vi "R4DataCollection.vi"(8 "error constant":errorcluster, 10 "Write Once":bool, 11 "LabVIEW Web Service":refnum<class "Web Service.lvclass">) -> (0 "error out":errorcluster={"status"=FALSE, "code"=0, "source"="0"})   [LabVIEW 2016]
uses:
  <vilib>/wsapi/Web Service.lvclass
  <vilib>/Platform/TimedLoop/XDataNode/timing_clust.ctl
  <vilib>/Platform/TimedLoop/XDataNode/nitl_modes.ctl
  <vilib>/Platform/TimedLoop/XDataNode/wakeup.ctl
  <vilib>/Platform/TimedLoop/XDataNode/XDataNode.xnode
  <vilib>/Platform/TimedLoop/XDataNode/XDNodeRunTimeDep.lvlib
  <vilib>/ptbypt/NI_PtbyPt.lvlib
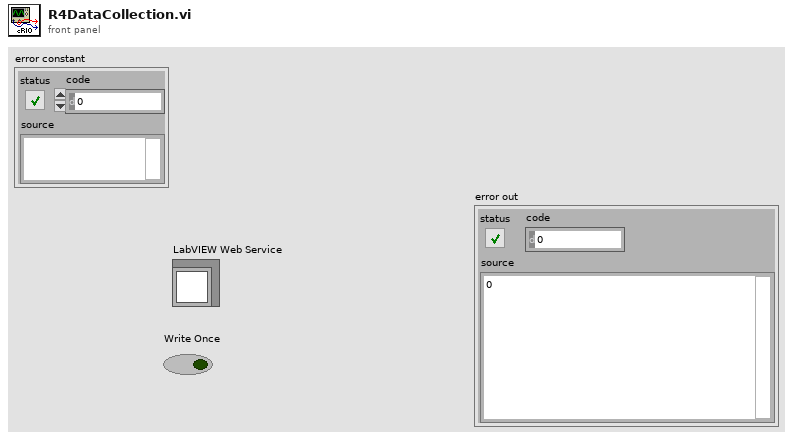
[diagram p1: front panel]
types:
  T1 = typedef "XDNodeRunTimeDep.lvlib/timing_clust.ctl" = cluster{"Expected End [f-1]":u64, "Actual End [f-1]":u64, "Finished Late? [f-1]":bool, "Expected End [i-1]":u64, "Actual End [i-1]":u64, "Finished Late? [i-1]":bool, "Expected Start [i]":u64, "Actual Start [i]":u64, "Expected Start [f]":u64, "Actual Start [f]":u64, "Source Name":string, "Structure Name":string, "Period":i64, "Deadline":i64, "Offset":i64, "Start":i64, "Priority":i32, "Timeout":i32, "Mode":T2, "Wakeup Reason":T3, "Error":errorcluster, "Source Type":string, "Secondary Source Type":string, "Global End Time":u64, "Global Start Time":u64, "Frame Duration":u64, "Iteration Duration":u64, "Assigned CPU":i32, "I/O Scan Engine Mode":u32}
  T2 = typedef "XDNodeRunTimeDep.lvlib/nitl_modes.ctl" = enum32{"No Change", "Process missed periods, maintain original phase", "Discard missed periods, maintain original phase", "Process missed periods, ignore original phase", "Discard missed periods, ignore original phase"}
  T3 = typedef "XDNodeRunTimeDep.lvlib/wakeup.ctl" = enum32{"Normal", "Aborted", "Asynchronous wakeup", "Timing source error", "Timed loop error", "Timeout"}
  T4 = cluster{"Media Pump":bool, "Water Pump":bool, "Gas Pump":bool, "Effluent Pump":bool, "Release Pump":bool}
  T5 = cluster{"Array of Double[0]":dbl, "Array of Double[1]":dbl, "Array of Double[2]":dbl, "Array of Double[3]":dbl, "Array of Double[4]":dbl, "Array of Double[5]":dbl, "Array of Double[6]":dbl, "Array of Double[7]":dbl, "Array of Double[8]":dbl}
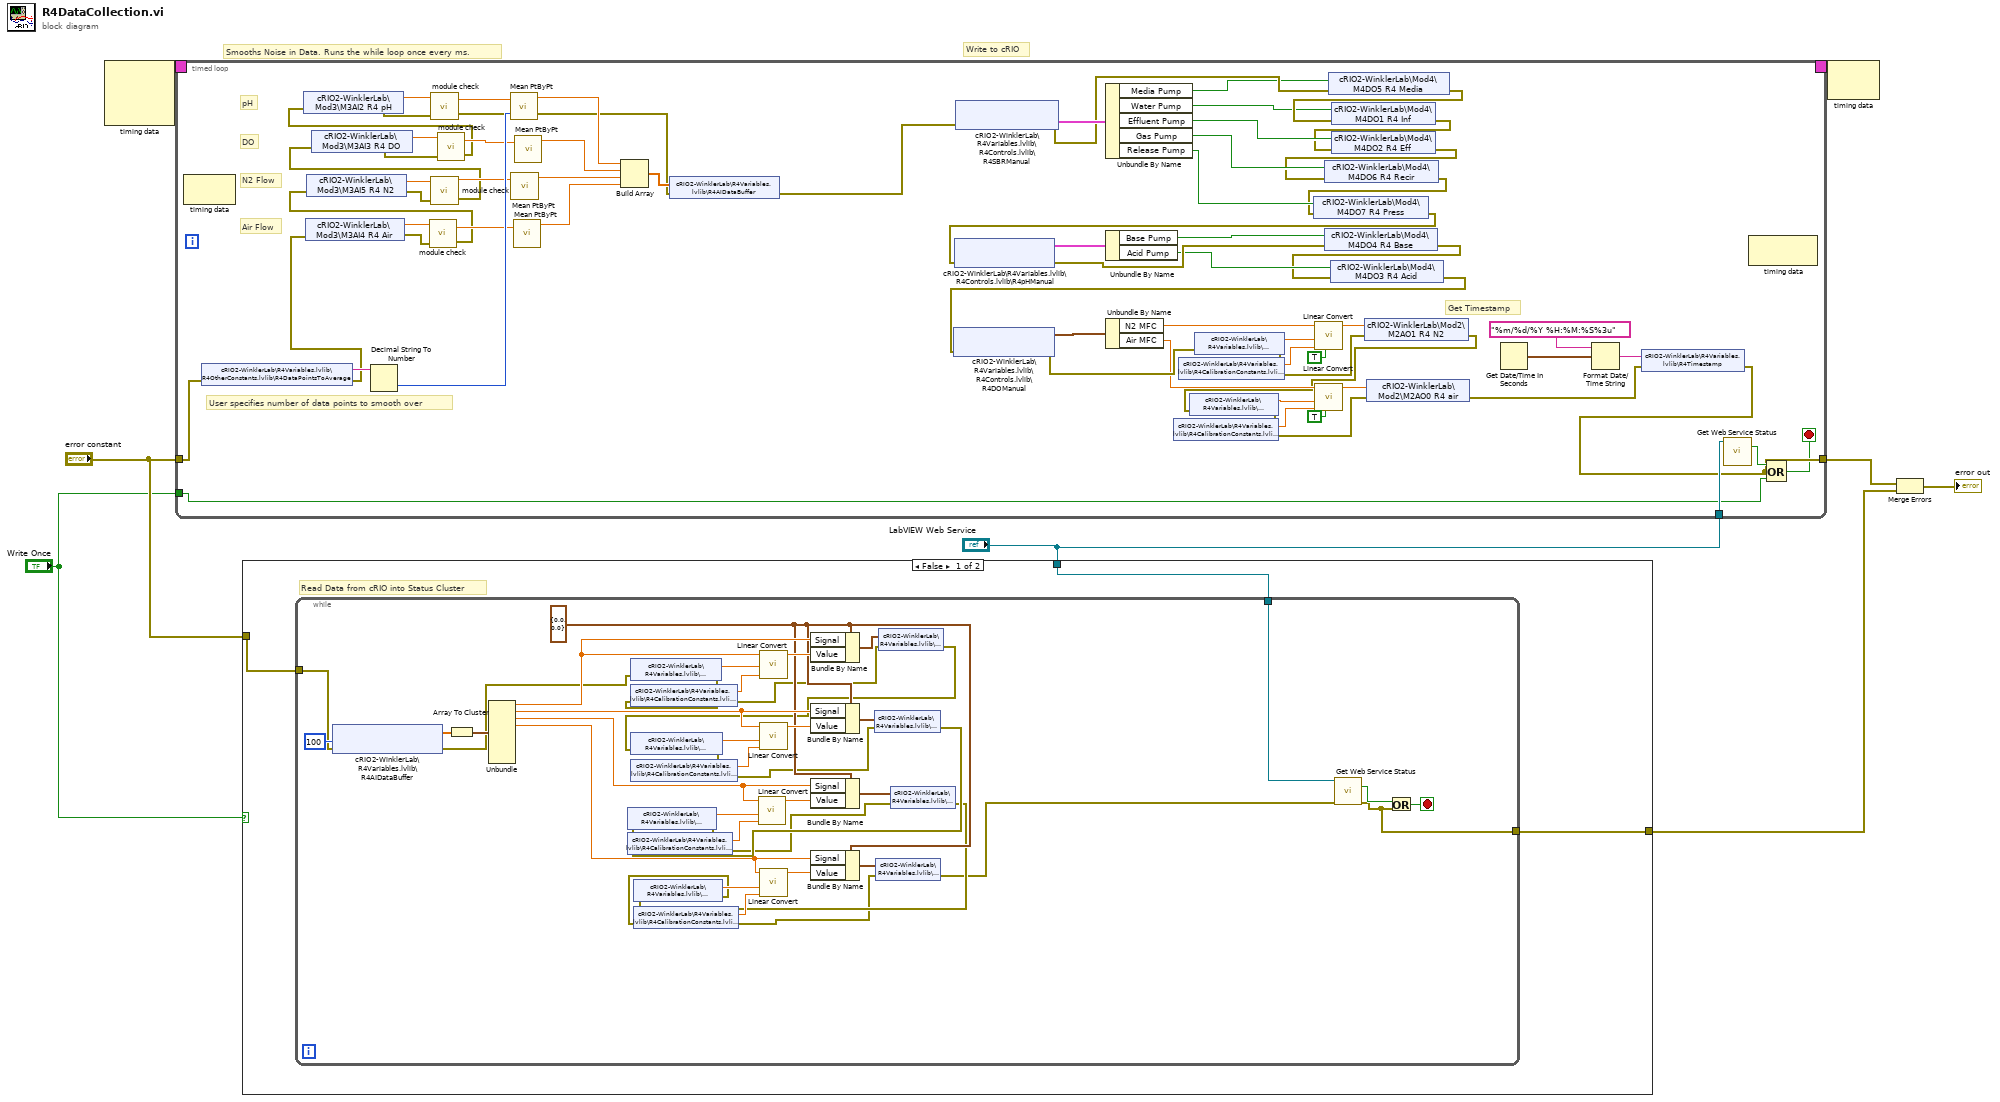
[diagram p0: block diagram]
diagram:
  # "Write to cRIO"
  # "Smooths Noise in Data. Runs the while loop once every ms."
  n1 = node-c288() -> (w8:T1)  [unwired: 3 in]
  n2 = timed-loop {
    timing: w8 -> [_]
    timing-out: [_] -> w7
    tunnel: "error constant" -> [w71]
    tunnel: "LabVIEW Web Service" -> [w67]
    tunnel: "Write Once" -> [w65]
    tunnel: [w64] -> w3
    stop <- w63 stop-if-true
    # "Get Timestamp"
    # "User specifies number of data points to smooth over"
    # "Air Flow"
    # "N2 Flow"
    # "DO"
    # "pH"
    n3 = node-c288() -> ()  [unwired: 1 in, 1 out]
    n4 = shared-variable "cRIO2-WinklerLab\\R4Variables.lvlib\\R4OtherConstants.lvlib\\R4DataPointsToAverage"(error in=w71) -> (w74:string, error out=w47:errorcluster)
    n5 = shared-variable "cRIO2-WinklerLab\\Mod3\\M3AI4 R4 Air"(error in=w47) -> (w13:dbl, error out=w12:errorcluster)
    n6 = Decimal String To Number(string=w74) -> (number=w62:i32)  [unwired: 2 in, 1 out]
    n7 = call "module check.vi"("error in"=w12, "Value"=w13) -> ("error constant"=w14:errorcluster, "Value out"=w15:dbl)  [unwired: 1 in]
    n8 = shared-variable "cRIO2-WinklerLab\\Mod3\\M3AI5 R4 N2"(error in=w14) -> (w17:dbl, error out=w16:errorcluster)
    n9 = call "module check.vi"("error in"=w16, "Value"=w17) -> ("error constant"=w18:errorcluster, "Value out"=w19:dbl)  [unwired: 1 in]
    n10 = shared-variable "cRIO2-WinklerLab\\Mod3\\M3AI3 R4 DO"(error in=w18) -> (w21:dbl, error out=w20:errorcluster)
    n11 = call "module check.vi"("error in"=w20, "Value"=w21) -> ("error constant"=w22:errorcluster, "Value out"=w23:dbl)  [unwired: 1 in]
    n12 = shared-variable "cRIO2-WinklerLab\\Mod3\\M3AI2 R4 pH"(error in=w22) -> (w26:dbl, error out=w24:errorcluster)
    n13 = call "module check.vi"("error in"=w24, "Value"=w26) -> ("error constant"=w25:errorcluster, "Value out"=w27:dbl)  [unwired: 1 in]
    n14 = call <vilib>:"Mean PtByPt.vi"("x"=w27, "sample length"=w62) -> ("mean"=w61:dbl)  [unwired: 2 in, 1 out]
    n15 = call <vilib>:"Mean PtByPt.vi"("x"=w19) -> ("mean"=w59:dbl)  [unwired: 3 in, 1 out]
    n16 = call <vilib>:"Mean PtByPt.vi"("x"=w15) -> ("mean"=w60:dbl)  [unwired: 3 in, 1 out]
    n17 = call <vilib>:"Mean PtByPt.vi"("x"=w23) -> ("mean"=w58:dbl)  [unwired: 3 in, 1 out]
    n18 = Build Array(w61, w58, w59, w60) -> (w78:dbl[])
    n19 = shared-variable "cRIO2-WinklerLab\\R4Variables.lvlib\\R4AIDataBuffer"(w78, error in=w25) -> (error out=w70:errorcluster)
    n20 = shared-variable "cRIO2-WinklerLab\\R4Variables.lvlib\\R4Controls.lvlib\\R4SBRManual"(error in=w70) -> (w73:T4, error out=w46:errorcluster)  [unwired: 1 in, 1 out]
    n21 = Unbundle By Name(w73) -> ("Media Pump"=w45:bool, "Water Pump"=w43:bool, "Effluent Pump"=w42:bool, "Gas Pump"=w40:bool, "Release Pump"=w11:bool)
    n22 = shared-variable "cRIO2-WinklerLab\\Mod4\\M4DO5 R4 Media"(w45, error in=w46) -> (error out=w44:errorcluster)
    n23 = shared-variable "cRIO2-WinklerLab\\Mod4\\M4DO1 R4 Inf"(w43, error in=w44) -> (error out=w41:errorcluster)
    n24 = shared-variable "cRIO2-WinklerLab\\Mod4\\M4DO2 R4 Eff"(w42, error in=w41) -> (error out=w39:errorcluster)
    n25 = shared-variable "cRIO2-WinklerLab\\Mod4\\M4DO6 R4 Recir"(w40, error in=w39) -> (error out=w10:errorcluster)
    n26 = shared-variable "cRIO2-WinklerLab\\Mod4\\M4DO7 R4 Press"(w11, error in=w10) -> (error out=w9:errorcluster)
    n27 = shared-variable "cRIO2-WinklerLab\\R4Variables.lvlib\\R4Controls.lvlib\\R4pHManual"(error in=w9) -> (w72:cluster{"Acid Pump":bool, "Base Pump":bool}, error out=w37:errorcluster)  [unwired: 1 in, 1 out]
    n28 = Unbundle By Name(w72) -> ("Base Pump"=w38:bool, "Acid Pump"=w36:bool)
    n29 = shared-variable "cRIO2-WinklerLab\\Mod4\\M4DO4 R4 Base"(w38, error in=w37) -> (error out=w35:errorcluster)
    n30 = shared-variable "cRIO2-WinklerLab\\Mod4\\M4DO3 R4 Acid"(w36, error in=w35) -> (error out=w34:errorcluster)
    n31 = shared-variable "cRIO2-WinklerLab\\R4Variables.lvlib\\R4Controls.lvlib\\R4DOManual"(error in=w34) -> (w69:cluster{"Air MFC":dbl, "N2 MFC":dbl}, error out=w68:errorcluster)  [unwired: 1 in, 1 out]
    n32 = Unbundle By Name(w69) -> ("N2 MFC"=w57:dbl, "Air MFC"=w56:dbl)
    n33 = shared-variable "cRIO2-WinklerLab\\R4Variables.lvlib\\R4CalibrationConstants.lvlib\\R4N2Slope"(error in=w68) -> (w51:dbl, error out=w49:errorcluster)
    n34 = shared-variable "cRIO2-WinklerLab\\R4Variables.lvlib\\R4CalibrationConstants.lvlib\\R4N2Intercept"(error in=w49) -> (w50:dbl, error out=w30:errorcluster)
    n35 = call "Linear Convert.vi"("Inverse?"=TRUE, "Intercept"=w50, "Slope"=w51, "Signal"=w57) -> ("Result"=w29:dbl)  [unwired: 7 in]
    n36 = shared-variable "cRIO2-WinklerLab\\Mod2\\M2AO1 R4 N2"(w29, error in=w30) -> (error out=w28:errorcluster)
    n37 = shared-variable "cRIO2-WinklerLab\\R4Variables.lvlib\\R4CalibrationConstants.lvlib\\R4AirSlope"(error in=w28) -> (w53:dbl, error out=w48:errorcluster)
    n38 = shared-variable "cRIO2-WinklerLab\\R4Variables.lvlib\\R4CalibrationConstants.lvlib\\R4AirIntercept"(error in=w48) -> (w52:dbl, error out=w32:errorcluster)
    n39 = call "Linear Convert.vi"("Inverse?"=TRUE, "Intercept"=w52, "Slope"=w53, "Signal"=w56) -> ("Result"=w31:dbl)  [unwired: 7 in]
    n40 = shared-variable "cRIO2-WinklerLab\\Mod2\\M2AO0 R4 air"(w31, error in=w32) -> (error out=w33:errorcluster)
    n41 = Get Date/Time In Seconds() -> (seconds since 1Jan1904=w76:timestamp)
    n42 = Format Date/Time String(time format string (%c)="%m/%d/%Y %H:%M:%S%3u", seconds (now)=w76) -> (date/time string=w75:string)  [unwired: 1 in]
    n43 = shared-variable "cRIO2-WinklerLab\\R4Variables.lvlib\\R4Timestamp"(w75, error in=w33) -> (error out=w64:errorcluster)
    n44 = call <vilib>:"Get Web Service Status.vi"("LabVIEW Web Service"=w67) -> ("service stopping?"=w66:bool)  [unwired: 12 in, 2 out]
    n45 = node-c288() -> ()  [unwired: 1 in, 1 out]
    n46 = Compound Arithmetic op=OR(w66, w64, w65) -> (w63:bool)
  }
  n47 = case shown="False" "Write Once" {
    tunnel: "error constant" -> [w83 w126]
    tunnel: "LabVIEW Web Service" -> [w82 _]
    tunnel: [w81 w126] -> w2
    frame False {
      # "Read Data from cRIO into Status Cluster"
      n48 = while {
        tunnel: w83 -> [w90]
        tunnel: [w89] -> w81
        tunnel: w82 -> [w88]
        stop <- w116 stop-if-true
        w107 = cluster{"Signal":dbl, "Value":dbl} {"Signal"=0.0, "Value"=0.0} ("Analog Input")
        n49 = shared-variable "cRIO2-WinklerLab\\R4Variables.lvlib\\R4AIDataBuffer"(error in=w90, u32 100 ("milliseconds to wait")) -> (w123:dbl[], error out=w100:errorcluster)  [unwired: 1 out]
        n50 = Array To Cluster(array=w123) -> (cluster=w125:T5)
        n51 = Unbundle(w125) -> ("Array of Double[0]"=w121:dbl, "Array of Double[1]"=w120:dbl, "Array of Double[2]"=w109:dbl, "Array of Double[3]"=w108:dbl)  [unwired: 5 out]
        n52 = shared-variable "cRIO2-WinklerLab\\R4Variables.lvlib\\R4CalibrationConstants.lvlib\\R4pHSlope"(error in=w100) -> (w114:dbl, error out=w99:errorcluster)
        n53 = shared-variable "cRIO2-WinklerLab\\R4Variables.lvlib\\R4CalibrationConstants.lvlib\\R4pHIntercept"(error in=w99) -> (w115:dbl, error out=w85:errorcluster)
        n54 = call "Linear Convert.vi"("Intercept"=w115, "Slope"=w114, "Signal"=w121) -> ("Result"=w122:dbl)  [unwired: 8 in]
        n55 = Bundle By Name(cluster=w107, "Signal"=w121, "Value"=w122) -> (w86:cluster{"Signal":dbl, "Value":dbl})
        n56 = shared-variable "cRIO2-WinklerLab\\R4Variables.lvlib\\R4Signals.lvlib\\R4pH"(w86, error in=w85) -> (error out=w87:errorcluster)
        n57 = shared-variable "cRIO2-WinklerLab\\R4Variables.lvlib\\R4CalibrationConstants.lvlib\\R4DOSlope"(error in=w87) -> (w113:dbl, error out=w98:errorcluster)
        n58 = shared-variable "cRIO2-WinklerLab\\R4Variables.lvlib\\R4CalibrationConstants.lvlib\\R4DOIntercept"(error in=w98) -> (w112:dbl, error out=w97:errorcluster)
        n59 = call "Linear Convert.vi"("Intercept"=w112, "Slope"=w113, "Signal"=w120) -> ("Result"=w118:dbl)  [unwired: 8 in]
        n60 = Bundle By Name(cluster=w107, "Signal"=w120, "Value"=w118) -> (w119:cluster{"Signal":dbl, "Value":dbl})
        n61 = shared-variable "cRIO2-WinklerLab\\R4Variables.lvlib\\R4Signals.lvlib\\R4DO"(w119, error in=w97) -> (error out=w96:errorcluster)
        n62 = shared-variable "cRIO2-WinklerLab\\R4Variables.lvlib\\R4CalibrationConstants.lvlib\\R4N2Slope"(error in=w96) -> (w104:dbl, error out=w95:errorcluster)
        n63 = shared-variable "cRIO2-WinklerLab\\R4Variables.lvlib\\R4CalibrationConstants.lvlib\\R4N2Intercept"(error in=w95) -> (w103:dbl, error out=w94:errorcluster)
        n64 = call "Linear Convert.vi"("Intercept"=w103, "Slope"=w104, "Signal"=w109) -> ("Result"=w110:dbl)  [unwired: 8 in]
        n65 = Bundle By Name(cluster=w107, "Signal"=w109, "Value"=w110) -> (w101:cluster{"Signal":dbl, "Value":dbl})
        n66 = shared-variable "cRIO2-WinklerLab\\R4Variables.lvlib\\R4Signals.lvlib\\R4N2"(w101, error in=w94) -> (error out=w93:errorcluster)
        n67 = shared-variable "cRIO2-WinklerLab\\R4Variables.lvlib\\R4CalibrationConstants.lvlib\\R4AirSlope"(error in=w93) -> (w106:dbl, error out=w92:errorcluster)
        n68 = shared-variable "cRIO2-WinklerLab\\R4Variables.lvlib\\R4CalibrationConstants.lvlib\\R4AirIntercept"(error in=w92) -> (w105:dbl, error out=w91:errorcluster)
        n69 = call "Linear Convert.vi"("Intercept"=w105, "Slope"=w106, "Signal"=w108) -> ("Result"=w111:dbl)  [unwired: 8 in]
        n70 = Bundle By Name(cluster=w107, "Signal"=w108, "Value"=w111) -> (w102:cluster{"Signal":dbl, "Value":dbl})
        n71 = shared-variable "cRIO2-WinklerLab\\R4Variables.lvlib\\R4Signals.lvlib\\R4Air"(w102, error in=w91) -> (error out=w84:errorcluster)
        n72 = call <vilib>:"Get Web Service Status.vi"("LabVIEW Web Service"=w88, "error in (no error)"=w84) -> ("service stopping?"=w117:bool, "error out"=w89:errorcluster)  [unwired: 11 in, 1 out]
        n73 = Or(x=w117, y=w89) -> (x .or. y?=w116:bool)
      }
    }
    frame True {
    }
  }
  n74 = node-c288(w7) -> ()  [unwired: 1 out]
  n75 = Merge Errors(w3, w2) -> (→"error out":errorcluster)
